vi "Run Test.vi"(8 "error in (no error)":errorcluster, 11 "Measurement in":refnum<class "Measurement.lvclass">) -> (0 "error out":errorcluster, 1 "Positions":i32[](array[numeric]), 2 "Tests Passed":bool[](array[boolean]), 3 "Measurement out":refnum<class "Measurement.lvclass">, 5 "Fail Codes":string[](array[string]))   [LabVIEW 2015, in "Measurement.lvclass"]
uses:
  Measurement.lvclass
  Test Class/Test Class.lvclass
  Classes/Application/Class/Application.lvclass
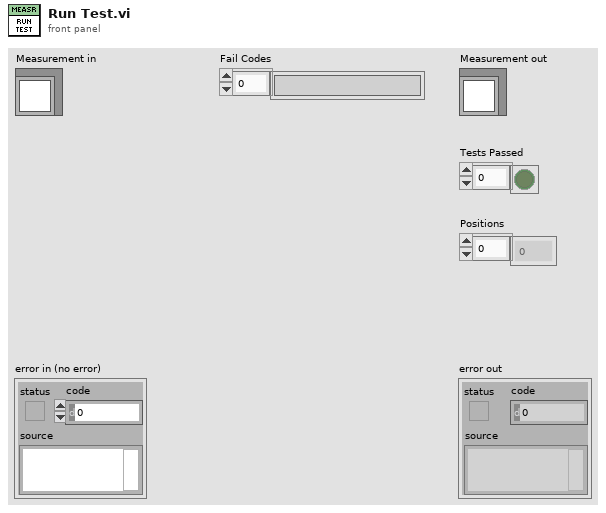
[diagram p1: front panel]
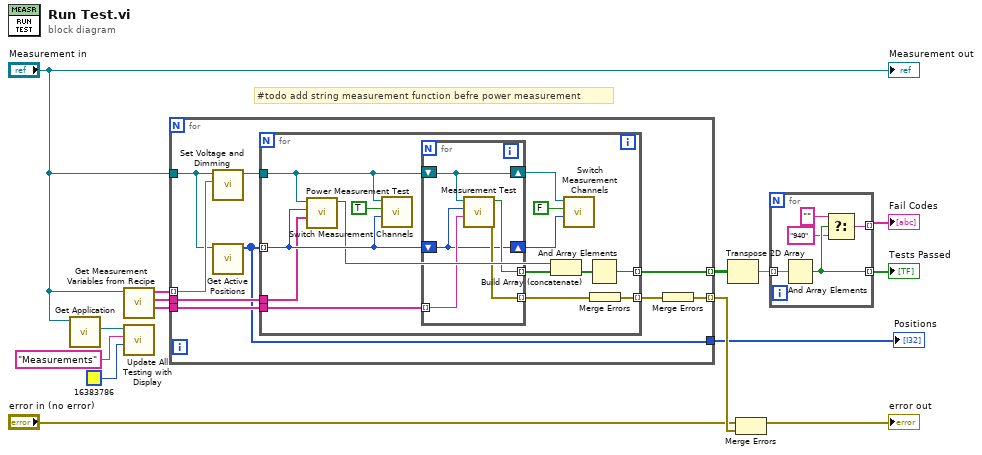
[diagram p0: block diagram]
diagram:
  # "#todo add string measurement function befre power measurement"
  n1 = call "Get Application.vi"("Test Class in"="Measurement in") -> ("Application.lvlib:Application.lvclass"=w5:refnum<class "Application.lvclass">)  [unwired: 9 in, 1 out]
  n2 = call "Get Measurement Variables from Recipe.vi"("Measurement in"="Measurement in") -> ("Measurements"=w2:string[], "Power Measurements"=w8:string[], "Measurement Voltages"=w9:string[])  [unwired: 7 in, 1 out]
  n3 = call "Update All Testing with Display.vi"("BG Color"=u32 16383786, "Message ('')"="Measurements", "Application in"=w5) -> ()  [unwired: 7 in, 2 out]
  n4 = for {
    tunnel: "Measurement in" -> [w20]
    tunnel: [w24] -> w15 mode=indexing
    tunnel: [w22] -> w12 mode=indexing
    tunnel: w9 -> [w21] mode=indexing
    tunnel: w8 -> [w17]
    tunnel: w2 -> [w18]
    tunnel: [w16] -> w1
    n5 = call "Set Voltage and Dimming.vi"("Measurement Voltage"=w21, "Measurement in"=w20) -> ("Measurement out"=w19:refnum<class "Measurement.lvclass">)  [unwired: 8 in, 1 out]
    n6 = call "Get Active Positions.vi"("Test Class in"=w20) -> ("Active Positions"=w16:u32[])  [unwired: 9 in, 1 out]
    n7 = for {
      tunnel: w16 -> [w28] mode=indexing
      tunnel: [w37] -> w24 mode=indexing
      tunnel: [w34] -> w23 mode=indexing
      tunnel: w19 -> [w29]
      tunnel: w18 -> [w30]
      tunnel: w17 -> [w27]
      n8 = call "Power Measurement Test.vi"("Power Measurements"=w27, "Position"=w28, "Measurement in"=w29) -> ("Passed"=w25:bool)  [unwired: 7 in, 1 out]
      n9 = call "Switch Measurement Channels.vi"("Position"=w28, "Switch On?"=TRUE, "Measurement in"=w29) -> ()  [unwired: 8 in, 1 out]
      n10 = for {
        tunnel: [w41] -> w38 mode=indexing
        tunnel: [w42] -> w35 mode=indexing
        tunnel: w30 -> [w43] mode=indexing
        shift-right: [w40] -> w31
        shift-left: w28 -> [w40]
        shift-right: [w39] -> w32
        shift-left: w29 -> [w39]
        n11 = call "Measurement Test.vi"("Channel"=w43, "Position"=w40, "Measurement"=w39) -> ("error out"=w42:errorcluster, "Passed"=w41:bool)  [unwired: 7 in]
      }
      n12 = Build Array (concatenate)(w25, w38) -> (w26:bool[])
      n13 = call "Switch Measurement Channels.vi"("Position"=w31, "Switch On?"=FALSE, "Measurement in"=w32) -> ()  [unwired: 8 in, 1 out]
      n14 = And Array Elements(Boolean array=w26) -> (logical AND=w37:bool)
      n15 = Merge Errors(w35) -> (w34:errorcluster)
    }
    n16 = Merge Errors(w23) -> (w22:errorcluster)
  }
  "Positions" <- w1
  n17 = Transpose 2D Array(2D array=w15) -> (transposed array=w14:bool[][])
  n18 = Merge Errors("error in (no error)", w12) -> (→"error out":errorcluster)
  n19 = for {
    tunnel: w14 -> [w48] mode=indexing
    tunnel: [w46] -> w13 mode=indexing
    tunnel: [w45] -> w4 mode=indexing
    n20 = And Array Elements(Boolean array=w48) -> (logical AND=w45:bool)
    n21 = Select(t="", s=w45, f="940") -> (s? t:f=w46:string)
  }
  "Tests Passed" <- w4
  "Fail Codes" <- w13
  "Measurement out" <- "Measurement in"
